vi "open.vi"(8 "error in (no error)":errorcluster, 9 "file status flags (default: none)":T1[](array[typedef]) items=["O_NONBLOCK"=2048], 10 "file creation flags":T2[](array[typedef]) items=["O_RDONLY"=0, "O_WRONLY"=1, "O_RDWR"=2, "O_CREAT"=64, "O_EXCL"=128, "O_TRUNC"=512], 11 "pathname":string) -> (0 "error out":errorcluster, 3 "file descriptor":i32)   [LabVIEW 2016, in "Linux RT IPC.C.lvlib"]
uses:
  Linux RT IPC.C.lvlib
  Controls/file creation flags.ctl
  Controls/file status flags.ctl
  Controls/functions.ctl
  <vilib>/NI/NI Linux RT Errno/Linux Errno.lvlib
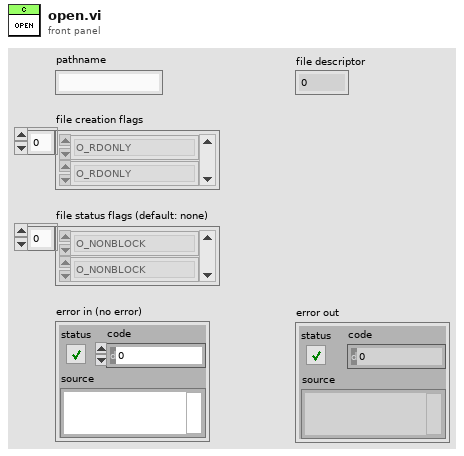
[diagram p1: front panel]
types:
  T1 = typedef "Linux RT IPC.C.lvlib/file status flags.ctl" = u32
  T2 = typedef "Linux RT IPC.C.lvlib/file creation flags.ctl" = u32
  T3 = typedef "Linux RT IPC.C.lvlib/functions.ctl" = enum16{"unspecified", "close", "epoll_create", "epoll_ctl", "epoll_wait", "fstat", "ftruncate", "mkfifo", "mmap", "munmap", "open", "read", "shm_open", "shm_unlink", "timerfd_create", "timerfd_settime", "timerfd_gettime", "write", "unlink"}
  T4 = typedef "Linux Errno.lvlib/errno.ctl" = enum16{"NO ERROR", "EPERM", "ENOENT", "ESRCH", "EINTR", "EIO", "ENXIO", "E2BIG", "ENOEXEC", "EBADF", "ECHILD", "EAGAIN", "ENOMEM", "EACCES", "EFAULT", "ENOTBLK", "EBUSY", "EEXIST", "EXDEV", "ENODEV", "ENOTDIR", "EISDIR", "EINVAL", "ENFILE", "EMFILE", "ENOTTY", "ETXTBSY", "EFBIG", "ENOSPC", "ESPIPE", "EROFS", "EMLINK", "EPIPE", "EDOM", "ERANGE", "EDADLK", "ENAMETOOLONG", "ENOLCK", "ENOSYS", "ENOTEMPTY", "ELOOP", "EWOULDBLOCK", "ENOMSG", "EIDRM", "ECHRNG", "EL2NSYNC", "EL3HLT", "EL3RST", "ELNRNG", "EUNATCH", "ENOCSI", "EL2HLT", "EBADE", "EBADR", "EXFULL", "ENOANO", "EBADRQC", "EBADSLT", "EDEADLOCK", "EBFONT", "ENOSTR", "ENODATA", "ETIME", "ENOSR", "ENONET", "ENOPKG", "EREMOTE", "ENOLINK", "EADV", "ESRMNT", "ECOMM", "EPROTO", "EMULTIHOP", "EDOTDOT", "EBADMSG", "EOVERFLOW", "ENOTUNIQ", "EBADFD", "EREMCHG", "ELIBACC", "ELIBBAD", "ELIBSCN", "ELIBMAX", "ELIBEXEC", "ELISEQ", "ERESTART", "ESTRPIPE", "EUSERS", "ENOTSOCK", "EDESTADDRREQ", "EMSGSIZE", "EPROTOTYPE", "ENOPROTOOPT", "EPROTONOSUPPORT", "ESOCKTNOSUPPORT", "EOPNOTSUPP", "EPFNOSUPPORT", "EAFNOSUPPORT", "EADDRINUSE", "EADDRNOTAVAIL", "ENETDOWN", "ENETUNREACH", "ENETRESET", "ECONNABORTED", "ECONNRESET", "ENOBUFS", "EISCONN", "ENOTCONN", "ESHUTDOWN", "ETOOMANYREFS", "ETIMEDOUT", "ECONNREFUSED", "EHOSTDOWN", "EHOSTUNREACH", "EALREADY", "EINPROGRESS", "ESTALE", "EUCLEAN", "ENOTNAM", "ENAVAIL", "EISNAM", "EREMOTEIO", "EDQUOT", "ENOMEDIUM", "EMEDIUMTYPE", "ECANCELED", "ENOKEY", "EKEYEXPIRED", "EKEYREVOKED", "EKEYREJECTED", "EOWNERDEAD", "ENOTRECOVERABLE", "ERFKILL", "EHWPOISON", "UNDEFINED"}
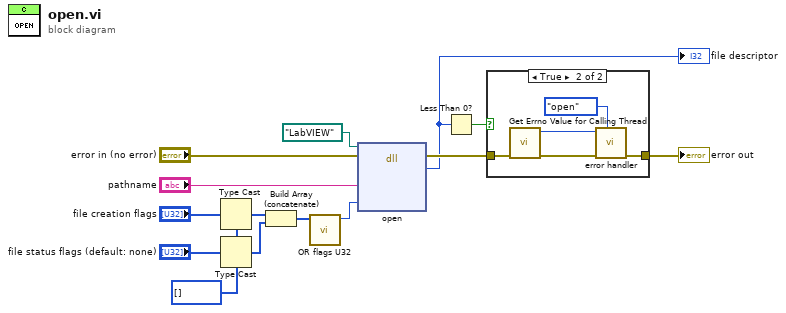
[diagram p0: block diagram]
diagram:
  w2 = u32[] []
  n1 = Type Cast(type=w2, x="file creation flags") -> (*(type *) &x=w4:u32[])
  n2 = Type Cast(type=w2, x="file status flags (default: none)") -> (*(type *) &x=w1:u32[])
  n3 = Build Array (concatenate)(w4, w1) -> (w6:u32[])
  n4 = call "OR flags U32.vi"("flags"=w6) -> ("OR'ed flags"=w7:u32)  [unwired: 10 in]
  n5 = dll-call lib="LabVIEW" fn="open"(path in=path "LabVIEW", error in="error in (no error)", "pathname"="pathname", "flags"=w7) -> (error out=w12:errorcluster, "return"=w8:i32)  [unwired: 3 in, 1 out]
  "file descriptor" <- w8
  n6 = Less Than 0?(x=w8) -> (x < 0?=w10:bool)
  n7 = case shown="True" w10 {
    tunnel: w12 -> [w15 w20]
    tunnel: [w15 w19] -> w11
    frame False {
    }
    frame True {
      n8 = call <vilib>:"Get Errno Value for Calling Thread.vi"("error in (no error)"=w20) -> ("error out"=w17:errorcluster, "errno"=w18:T4)  [unwired: 9 in]
      n9 = call "error handler.vi"("function (unspecified)"=functions."open" ("function"), "error in (no error)"=w17, "errno"=w18) -> ("error out"=w19:errorcluster)  [unwired: 8 in]
    }
  }
  "error out" <- w11
